vi "transform.vi"(8 "Error In":errorcluster, 11 "Input":sgl[][](array[numeric])) -> (0 "Error Out":errorcluster, 3 "Output":sgl[][](array[numeric]))   [LabVIEW 2014]
uses:
  UT FFTW States.ctl
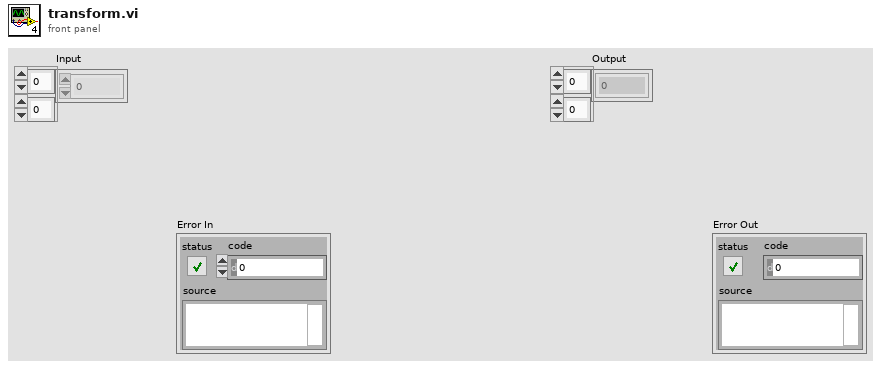
[diagram p1: front panel]
types:
  T1 = typedef "UT FFTW States.ctl" = enum16{"Init", "Transform", "Cleanup"}
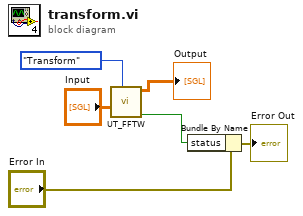
[diagram p0: block diagram]
diagram:
  n1 = call "UT_FFTW.vi"("UT FFTW States"=UT_FFTW_States."Transform", "Array"="Input") -> ("Error"=w1:bool, "Results"=→"Output":sgl[][])  [unwired: 8 in]
  n2 = Bundle By Name(cluster="Error In", "status"=w1) -> (→"Error Out":errorcluster)
